vi "Mouli_Softs.vi"(8 "entrée d'erreur":errorcluster, 9 "Branche":string="1", 11 "chemin":path) -> (0 "APPL":string, 1 "ESW":string, 2 "CONFIG":string, 3 "ASW":string)   [LabVIEW 2020]
uses:
  <vilib>/regexp/Match Regular Expression.xnode
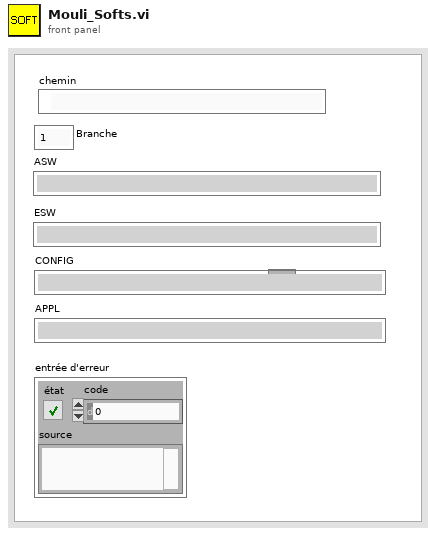
[diagram p1: front panel]
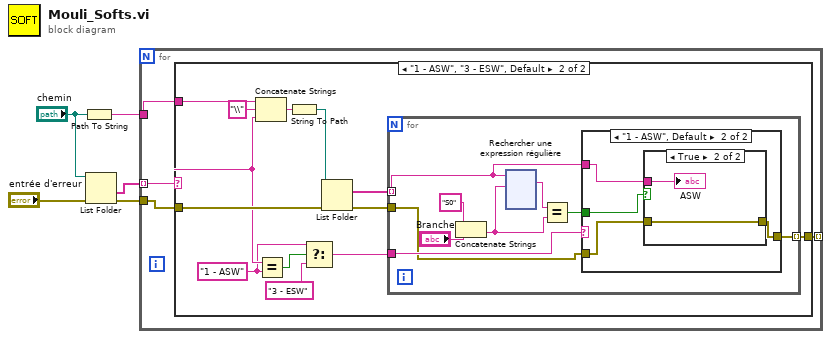
[diagram p0: block diagram]
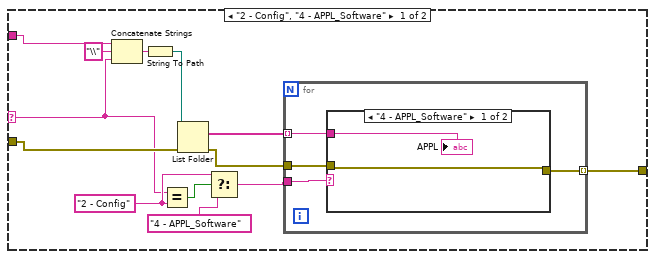
[diagram p2: hidden frame]
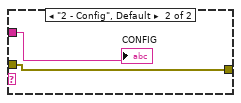
[diagram p3: hidden frame]
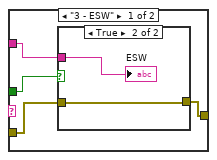
[diagram p4: hidden frame]
diagram:
  n1 = Path To String(path="chemin") -> (string=w4:string)
  n2 = List Folder(path="chemin", error in="entrée d'erreur") -> (folder names=w1:string[], error out=w2:errorcluster)  [unwired: 2 in, 2 out]
  n3 = for {
    tunnel: w4 -> [w9]
    tunnel: w1 -> [w7] mode=indexing
    tunnel: w2 -> [w8]
    tunnel: [w6] -> _ mode=indexing
    n4 = case shown="\"1 - ASW\", \"3 - ESW\", Default" w7 {
      selector: w7 -> [w14 w37]
      tunnel: w9 -> [w19 w43]
      tunnel: w8 -> [w18 w39]
      tunnel: [w10 w31] -> w6
      frame "2 - Config", "4 - APPL_Software" {
        w15 = "2 - Config"
        n5 = Concatenate Strings(w19, "\\" ("chaîne"), w14) -> (w21:string)
        n6 = String To Path(string=w21) -> (path=w20:path)
        n7 = Equal?(x=w14, y=w15) -> (x = y?=w17:bool)
        n8 = List Folder(path=w20, error in=w18) -> (filenames=w12:string[], error out=w11:errorcluster)  [unwired: 2 in, 2 out]
        n9 = Select(t=w15, s=w17, f="4 - APPL_Software") -> (s? t:f=w13:string)
        n10 = for {
          tunnel: w13 -> [w26]
          tunnel: w12 -> [w25] mode=indexing
          tunnel: [w24] -> w10 mode=indexing
          tunnel: w11 -> [w23]
          n11 = case shown="\"4 - APPL_Software\"" w26 {
            tunnel: w25 -> [w28 w30]
            tunnel: [w27 w29] -> w24
            tunnel: w23 -> [w27 w29]
            frame "4 - APPL_Software" {
              "APPL" <- w28
            }
            frame "2 - Config", Default {
              "CONFIG" <- w30
            }
          }
        }
      }
      frame "1 - ASW", "3 - ESW", Default {
        w34 = "1 - ASW"
        n12 = Concatenate Strings(w43, "\\" ("chaîne"), w37) -> (w41:string)
        n13 = Equal?(x=w37, y=w34) -> (x = y?=w36:bool)
        n14 = String To Path(string=w41) -> (path=w40:path)
        n15 = Select(t=w34, s=w36, f="3 - ESW") -> (s? t:f=w33:string)
        n16 = List Folder(path=w40, error in=w39) -> (filenames=w38:string[], error out=w32:errorcluster)  [unwired: 2 in, 2 out]
        n17 = for {
          tunnel: w38 -> [w49] mode=indexing
          tunnel: w33 -> [w48]
          tunnel: w32 -> [w46]
          tunnel: [w45] -> w31 mode=indexing
          n18 = Concatenate Strings("S0" ("chaîne"), "Branche") -> (w50:string)
          n19 = xnode "Rechercher une expression régulière"("chaîne en entrée"=w49, "expression régulière"=w50) -> ("toute l'expression"=w51:string)  [unwired: 4 in, 4 out]
          n20 = Equal?(x=w51, y=w50) -> (x = y?=w47:bool)
          n21 = case shown="\"1 - ASW\", Default" w48 {
            tunnel: w49 -> [w170 w177]
            tunnel: w47 -> [w169 w176]
            tunnel: w46 -> [w168 w175]
            tunnel: [w167 w174] -> w45
            frame "3 - ESW" {
              n22 = case shown="True" w169 {
                tunnel: w170 -> [_ w173]
                tunnel: [w171 w172] -> w167
                tunnel: w168 -> [w171 w172]
                frame False {
                }
                frame True {
                  "ESW" <- w173
                }
              }
            }
            frame "1 - ASW", Default {
              n23 = case shown="True" w176 {
                tunnel: w177 -> [_ w180]
                tunnel: w175 -> [w178 w179]
                tunnel: [w178 w179] -> w174
                frame False {
                }
                frame True {
                  "ASW" <- w180
                }
              }
            }
          }
        }
      }
    }
  }
